vi "UUIDs - Calculated Values v3.vi"(7 "Expressions":string[](array[string]), 8 "Error in":errorcluster, 10 "values in":dbl[](array[numeric]), 11 "UUIDs in":string[](array[string])) -> (0 "Error out":errorcluster, 2 "values out":dbl[](array[numeric])=[0.0, 999.0, 2.0, 3.0, nan, 5.0, 6.0, 7.0], 3 "UUIDs out":string[](array[string])=["A", "B", "C", "D", "E", "F", "G"])   [LabVIEW 2020]
doc: "Functional global variable. This VI calculates any configured UUIDs based on user-supplied formulas containing other UUIDs and numbers. Provides standard error functionality. UUIDs must not wholly contain other UUIDs for calculations to be parsed properly; i.e. \"Outlet Temp\" and \"Temp\" are incompatible UUIDs for this VI and any associated calculations will not be possible."
uses:
  <vilib>/gmath/NI_Gmath.lvlib
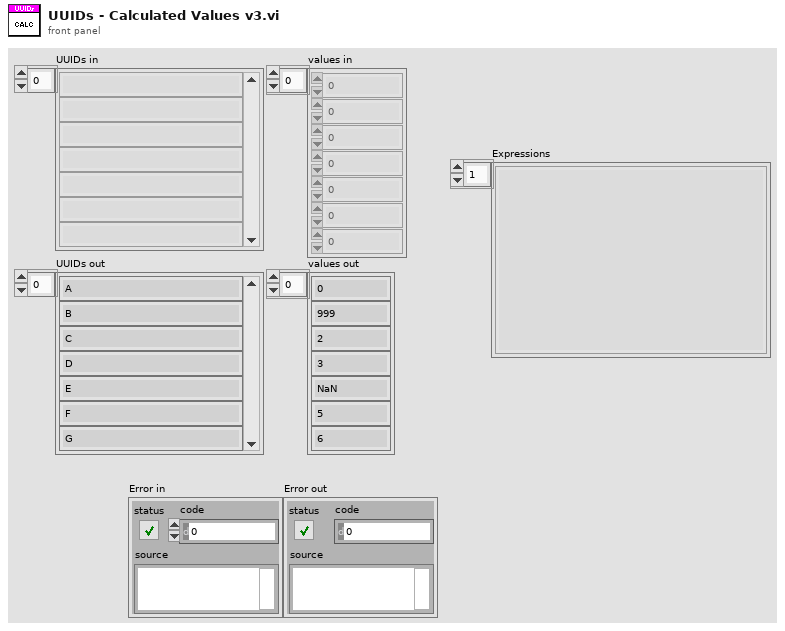
[diagram p1: front panel]
types:
  T1 = typedef "Tagged Calc Info.ctl" = cluster{"UUIDs":string[], "Calculated Channel Info":T2[]}
  T2 = typedef "UUIDs - Calculated Channel Info.ctl" = cluster{"Parsed Formula":cluster{"Table":i32[][], "Y Values":dbl[]}, "Formula UUIDs":string[], "Formula Variables":string[]}
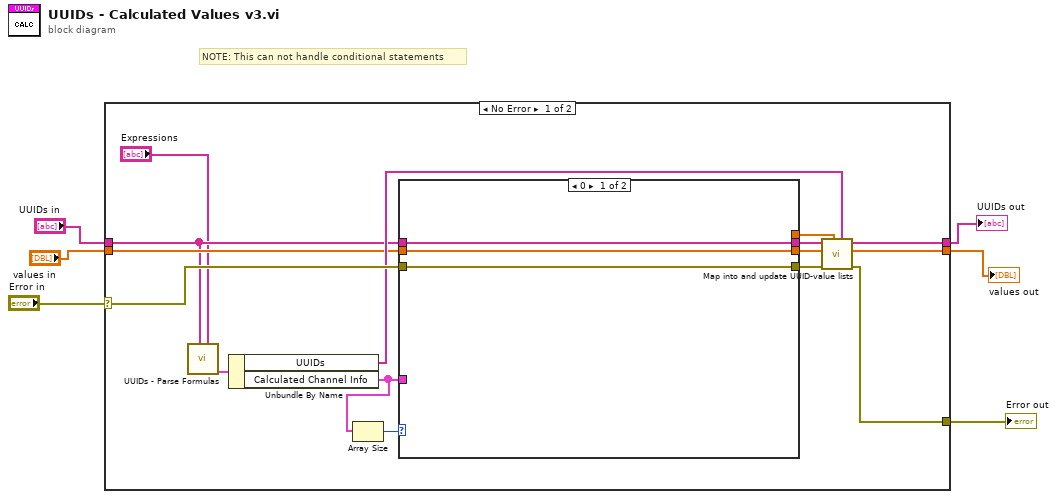
[diagram p0: block diagram]
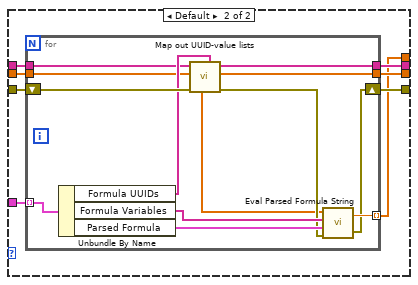
[diagram p2: hidden frame]
diagram:
  # "NOTE: This can not handle conditional statements"
  n1 = case shown="No Error" "Error in" {
    selector: "Error in" -> [w21 w48]
    tunnel: "UUIDs in" -> [w10 w47]
    tunnel: [w19 w48] -> w5
    tunnel: [w18 w47] -> w1
    tunnel: [w15 w46] -> w2
    tunnel: "values in" -> [w12 w46]
    frame No Error {
      n2 = call "UUIDs - Parse Formulas.vi"("Formulas"="Expressions", "All UUIDs"=w10) -> ("Tagged Calc Info"=w11:T1)  [unwired: 7 in]
      n3 = Unbundle By Name(w11) -> ("UUIDs"=w13:string[], "Calculated Channel Info"=w7:T2[])
      n4 = Array Size(array=w7) -> (size(s)=w8:i32)
      n5 = case shown="0" w8 {
        tunnel: w21 -> [w22 w32]
        tunnel: w7 -> [_ w31]
        tunnel: [w22 w30] -> w20
        tunnel: [w24 w29] -> w17
        tunnel: [w23 w28] -> w16
        tunnel: [_ w27] -> w14
        tunnel: w12 -> [w23 w26]
        tunnel: w10 -> [w24 w25]
        frame 0 {
        }
        frame Default {
          n6 = for {
            tunnel: w31 -> [w45] mode=indexing
            tunnel: [w42] -> w27 mode=indexing
            tunnel: [w39] -> w29
            tunnel: w25 -> [w38]
            tunnel: [w37] -> w28
            shift-right: [w35] -> w30
            shift-left: w32 -> [w41]
            tunnel: w26 -> [w34]
            n7 = Unbundle By Name(w45) -> ("Formula UUIDs"=w40:string[], "Formula Variables"=w44:string[], "Parsed Formula"=w43:cluster{"Table":i32[][], "Y Values":dbl[]})
            n8 = call "Map out UUID-value lists.vi"("UUIDs to extract"=w40, "error in"=w41, "values in"=w34, "UUIDs in"=w38) -> ("error out"=w36:errorcluster, "values out"=w37:dbl[], "UUIDs out"=w39:string[], "values extracted"=w33:dbl[])  [unwired: 3 in, 1 out]
            n9 = call <vilib>:"Eval Parsed Formula String.vi"("error in (no error)"=w36, "Parsed Formula"=w43, "Variables"=w44, "X Values"=w33) -> ("error out"=w35:errorcluster, "y value"=w42:dbl)
          }
        }
      }
      n10 = call "Map into and update UUID-value lists.vi"("UUIDs to replace"=w13, "values to replace"=w14, "error in"=w20, "values in"=w16, "UUIDs in"=w17) -> ("error out"=w19:errorcluster, "values out"=w15:dbl[], "UUIDs out"=w18:string[])  [unwired: 3 in, 1 out]
    }
    frame Error {
    }
  }
  "Error out" <- w5
  "values out" <- w2
  "UUIDs out" <- w1
